vi "写入V3.1外设配置.vi"(8 "error in (no error)":errorcluster, 10 "外设配置":T1 {"阀方向" items=["顺时针", "逆时针", "就近"]; "总氮x公式0" items=["0", "1"]; "光谱仪类型" items=["1型", "2型", "3型", "2型氙灯联控"]; "泵阀量" items=["9通"=9, "10通"=10, "12通"=12]; "泵类型" items=["1型", "2型", "sy04型+旋转阀"]}, 11 "MB session in":refnum<class "MB_Master.lvclass">) -> (0 "error out":errorcluster, 3 "MB session out":refnum<class "MB_Master.lvclass">)   [LabVIEW 2016, in "斯坦道氟化物.lvlib"]
uses:
  <vilib>/Plasmionique/MB Master/MB_Master/MB_Master.lvclass
  <vilib>/Plasmionique/MB Master/MB_Master_Serial/MB_Master_Serial.lvclass
  E:/Program Files (x86)/National Instruments/LabVIEW 2016/vi.lib/Plasmionique/MB Master/MB_Master/MB_Master.lvclass
  <vilib>/Plasmionique/MB Master/MB Master.lvlib
panel:
  in  "U32":u32
  in  "SGL":sgl
  in  "U16":u16
  in  "U8":u8
  in  "VISA Resource":refnum<visa-resource-name>
  in  "引用选择":enum16{"MB引用", "自建引用"}(ring)
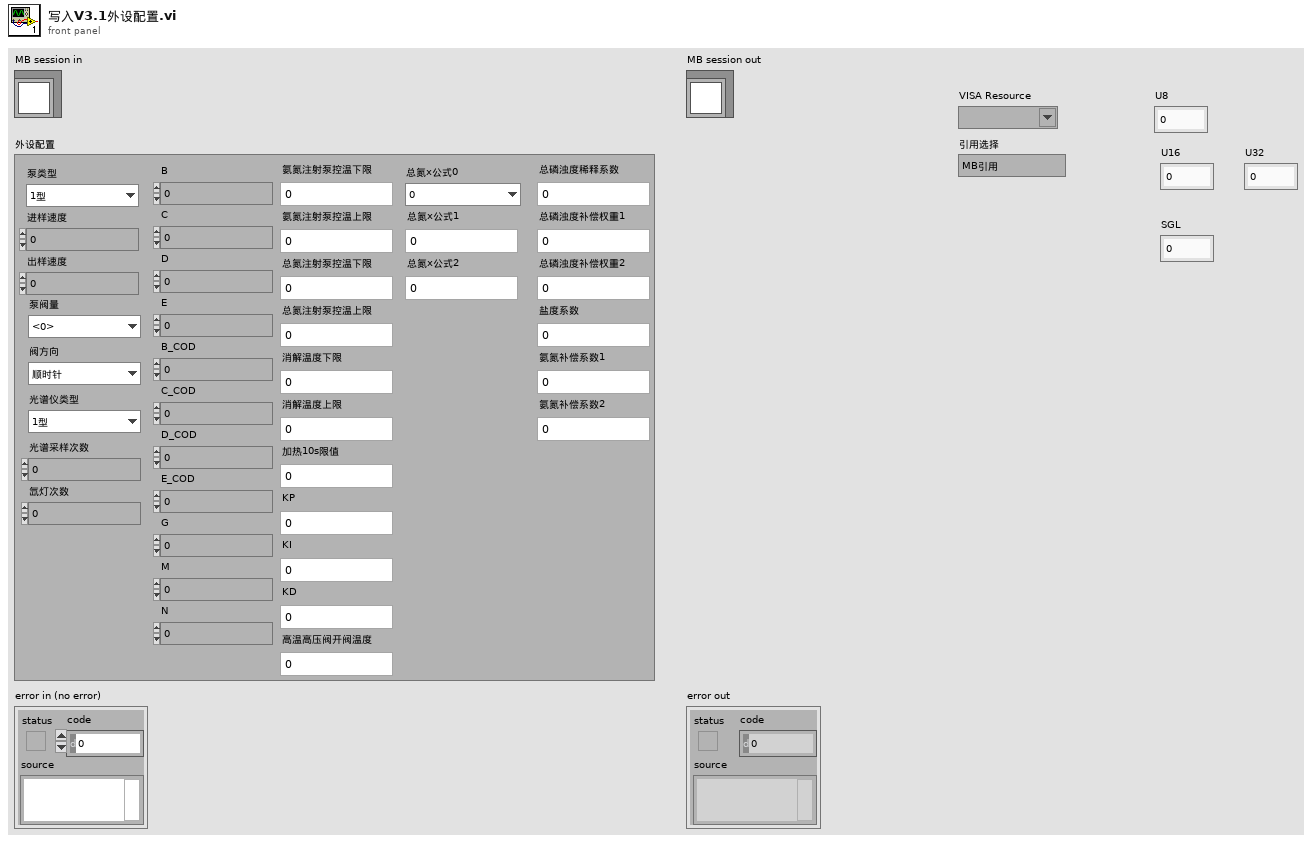
[diagram p1: front panel]
types:
  T1 = typedef "斯坦道氟化物.lvlib/V3.1版外设参数.ctl" = cluster{"泵类型":u8, "进样速度":u32, "出样速度":u32, "泵阀量":u8, "阀方向":u8, "光谱仪类型":u8, "光谱采样次数":u8, "氙灯次数":u8, "B":u16, "C":u16, "D":u16, "E":u16, "B_COD":u16, "C_COD":u16, "D_COD":u16, "E_COD":u16, "G":u16, "M":u16, "N":u16, "氨氮注射泵控温下限":sgl, "氨氮注射泵控温上限":sgl, "总氮注射泵控温下限":sgl, "总氮注射泵控温上限":sgl, "消解温度下限":sgl, "消解温度上限":sgl, "加热10s限值":sgl, "KP":sgl, "KI":sgl, "KD":sgl, "高温高压阀开阀温度":sgl, "总氮x公式0":u8, "总氮x公式1":sgl, "总氮x公式2":sgl, "总磷浊度稀释系数":sgl, "总磷浊度补偿权重1":sgl, "总磷浊度补偿权重2":sgl, "盐度系数":sgl, "氨氮补偿系数1":sgl, "氨氮补偿系数2":sgl}
  T2 = cluster{"baud rate (bps)":u32, "stop bits":u16, "parity":u16, "flow control":u16, "timeout":u32, "retries":i32}
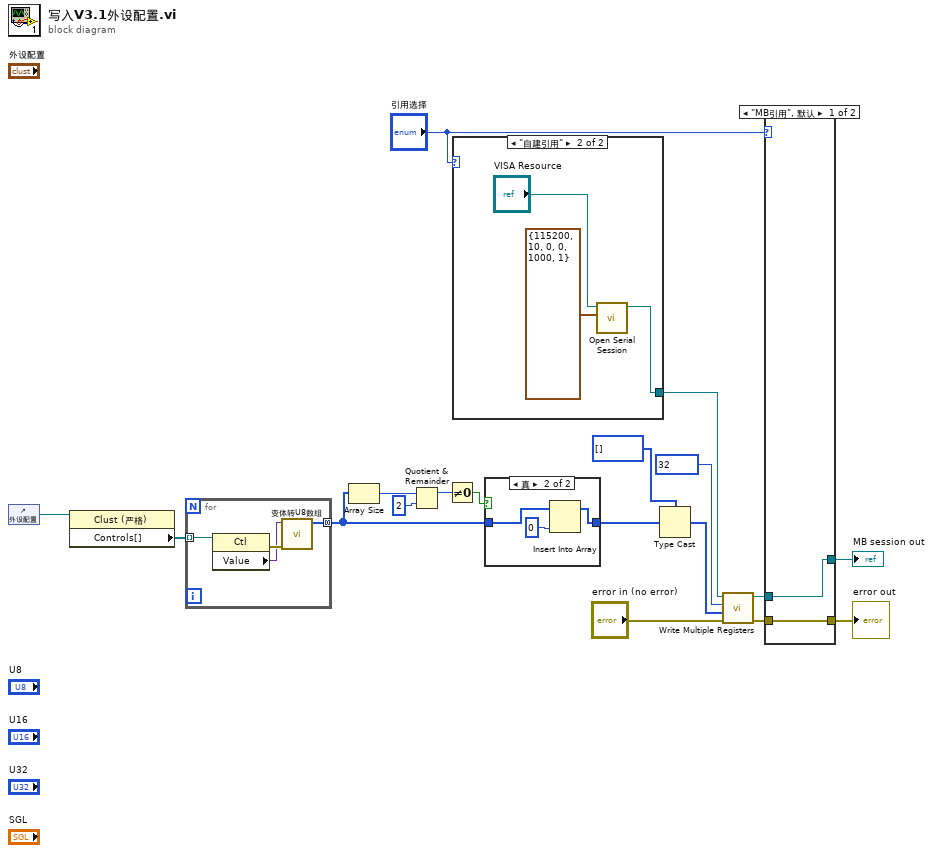
[diagram p0: block diagram]
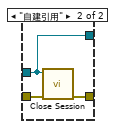
[diagram p3: hidden frame]
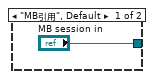
[diagram p4: hidden frame]
diagram:
  n1 = control-ref of="外设配置"() -> (w10:refnum<vi>)
  n2 = property class="Clust (严格)"(reference=w10) -> ("Controls[]"=w9:refnum<vi>[])  [unwired: 1 in, 2 out]
  n3 = for {
    tunnel: w9 -> [w22] mode=indexing
    tunnel: [w19] -> w2 mode=concatenating
    n4 = property class="Ctl"(reference=w22) -> (error out=w21:errorcluster, "Value"=w20:variant)  [unwired: 1 in, 1 out]
    n5 = call "变体转U8数组.vi"("错误输入（无错误）"=w21, "Value"=w20) -> ("U8数组"=w19:u8[])  [unwired: 8 in, 1 out]
  }
  n6 = Array Size(array=w2) -> (size(s)=w5:i32)
  n7 = Quotient & Remainder(x=w5, y=2) -> (x-y*floor(x/y)=w4:i32)  [unwired: 1 out]
  n8 = Not Equal To 0?(x=w4) -> (x != 0?=w3:bool)
  n9 = case shown="\"自建引用\"" "引用选择" {
    tunnel: ["MB session in" w26] -> w16
    frame "MB引用", Default {
    }
    frame "自建引用" {
      n10 = call <vilib>:"Open Serial Session.vi"("Serial Config"=T2 {"baud rate (bps)"=115200, "stop bits"=10, "parity"=0, "flow control"=0, "timeout"=1000, "retries"=1}, "VISA Resource"="VISA Resource") -> ("MB_Serial session"=w26:refnum<class "MB_Master_Serial.lvclass">)  [unwired: 8 in, 1 out]
    }
  }
  n11 = case shown="真" w3 {
    tunnel: w2 -> [w27 w30]
    tunnel: [w27 w28] -> w1
    frame False {
    }
    frame True {
      n12 = Insert Into Array(array=w30, new element=u8 0 ("新元素/子数组")) -> (w28:u8[])  [unwired: 1 in]
    }
  }
  n13 = Type Cast(type=u16[] [], x=w1) -> (*(type *) &x=w7:u16[])
  n14 = call <vilib>:"Write Multiple Registers.vi"("error in (no error)"="error in (no error)", "values"=w7, "starting address"=u16 32, "MB session in"=w16) -> ("error out"=w13:errorcluster, "MB session out"=w15:refnum<class "MB_Master.lvclass">)  [unwired: 6 in]
  n15 = case shown="\"MB引用\", 默认" "引用选择" {
    tunnel: w15 -> [w31 w33]
    tunnel: w13 -> [w32 w35]
    tunnel: [w32 w34] -> w12
    tunnel: [w31 w33] -> w11
    frame "MB引用", Default {
    }
    frame "自建引用" {
      n16 = call-dynamic "Close Session.vi"("error in (no error)"=w35, "MB session in"=w33) -> ("error out"=w34:errorcluster)  [unwired: 9 in]
    }
  }
  "MB session out" <- w11
  "error out" <- w12
